vi "Check Digital Pattern Name Collisions.vi"(4 "old name":string, 6 "old rio":string, 9 "new name":string, 10 "new rio":string, 11 "Patterns":T1[](array[typedef])) -> (2 "name collision?":bool, 3 "Patterns":T1[](array[typedef]))   [LabVIEW 2015, in "Engine Simulation Toolkit System Explorer.lvlib"]
uses:
  Engine Simulation Toolkit System Explorer.lvlib
  Digital Pattern.ctl
  Digital Pattern Base.ctl
  Digital Pattern Remove Edge.ctl
  Digital Pattern Add Pulse.ctl
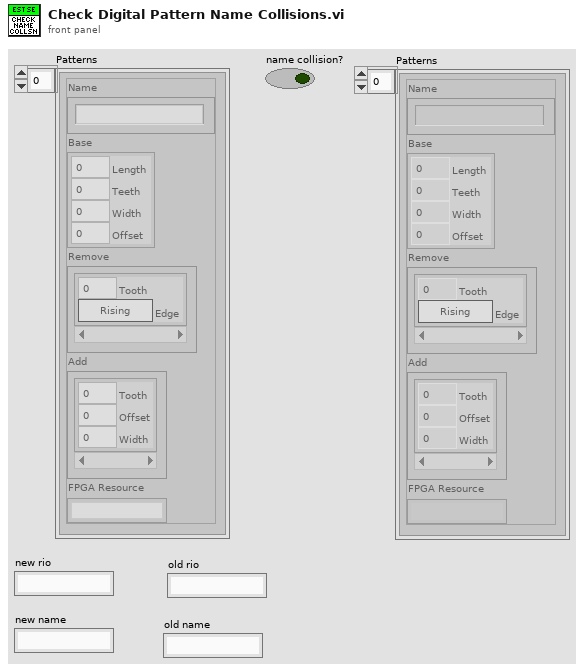
[diagram p1: front panel]
types:
  T1 = typedef "Engine Simulation Toolkit System Explorer.lvlib/Digital Pattern.ctl" = cluster{"Name":string, "Base":T2, "Remove":T3[], "Add":T4[], "FPGA Resource":string}
  T2 = typedef "Engine Simulation Toolkit System Explorer.lvlib/Digital Pattern Base.ctl" = cluster{"Length":dbl, "Teeth":u16, "Width":dbl, "Offset":dbl}
  T3 = typedef "Engine Simulation Toolkit System Explorer.lvlib/Digital Pattern Remove Edge.ctl" = cluster{"Tooth":u16, "Edge":bool}
  T4 = typedef "Engine Simulation Toolkit System Explorer.lvlib/Digital Pattern Add Pulse.ctl" = cluster{"Tooth":u16, "Offset":dbl, "Width":dbl}
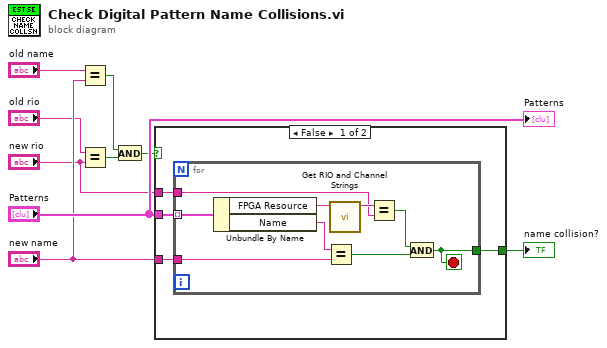
[diagram p0: block diagram]
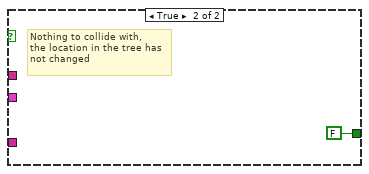
[diagram p2: hidden frame]
diagram:
  n1 = Equal?(x="old name", y="new name") -> (x = y?=w2:bool)
  n2 = Equal?(x="old rio", y="new rio") -> (x = y?=w3:bool)
  n3 = And(x=w2, y=w3) -> (x .and. y?=w1:bool)
  n4 = case shown="False" w1 {
    tunnel: "Patterns" -> [w13 _]
    tunnel: [w12 FALSE] -> w8
    tunnel: "new name" -> [w11 _]
    tunnel: "new rio" -> [w10 _]
    frame False {
      n5 = for {
        tunnel: w13 -> [w22] mode=indexing
        tunnel: w11 -> [w17]
        tunnel: w10 -> [w18]
        tunnel: [w14] -> w12
        stop <- w14 stop-if-true
        n6 = Unbundle By Name(w22) -> ("FPGA Resource"=w20:string, "Name"=w21:string)
        n7 = Equal?(x=w21, y=w17) -> (x = y?=w15:bool)
        n8 = call "Get RIO and Channel Strings.vi"("rio/channel"=w20) -> ("rio"=w19:string)  [unwired: 9 in, 1 out]
        n9 = Equal?(x=w19, y=w18) -> (x = y?=w16:bool)
        n10 = And(x=w16, y=w15) -> (x .and. y?=w14:bool)
      }
    }
    frame True {
      # "Nothing to collide with,\nthe location in the tree has\nnot changed"
    }
  }
  "name collision?" <- w8
  "Patterns" <- "Patterns"
